vi "ini_sesion.vi"(8 "error in (no error)":errorcluster, 11 "p2p vst in":refnum<class "p2p vst.lvclass">) -> (0 "error out":errorcluster, 3 "p2p vst out":refnum<class "p2p vst.lvclass">)   [LabVIEW 2021, in "p2p vst.lvclass"]
uses:
  p2p vst.lvclass
  p2p vst.lvclass/p2p vst.ctl
  <instrlib>/niRFSG/niRFSG.llb/niRFSG Ref Clock Sources.ctl
  <vilib>/FPGAPlugInAG/PXIe-5785 (KU060)/niLvFpga_Open_PXIe-5785 (KU060).vi
  <vilib>/rvi/interface/common/dynamic/niFpgaDynamicAddResources.vi
  <vilib>/FPGAPlugInAG/Dynamic/niLvFpga_P2PGetEndpoint_Dynamic.vi
  <vilib>/Utility/error.llb/Error Cluster From Error Code.vi
  <vilib>/rvi/interface/common/niFpgaWaitOnOcc.vi
  <vilib>/rvi/errors/niLvFpgaAdjustHostInterfaceError.vi
  <vilib>/rvi/interface/nirviOpenFPGA/nirviOpenFPGA.xnode
  FPGA Bitfiles/P2P_Pulse.lvbitx
  <vilib>/rvi/interface/nirviMethod/nirviMethod.xnode
  <vilib>/rvi/interface/nirviReadWriteControl/nirviReadWriteControl.xnode
  <vilib>/FPGAPlugInAG/Dynamic/niLvFpga_ConfigureFifo_Dynamic.vi
  <vilib>/rvi/errors/niLvFpgaMergeErrorWithErrorCode.vi
  <vilib>/FPGAPlugInAG/Dynamic/niLvFpga_StopFifo_Dynamic.vi
  NiFpgaLv.dll
  <vilib>/rvi/interface/Simulation/niFpgaSimulationCallBeginRW.vi
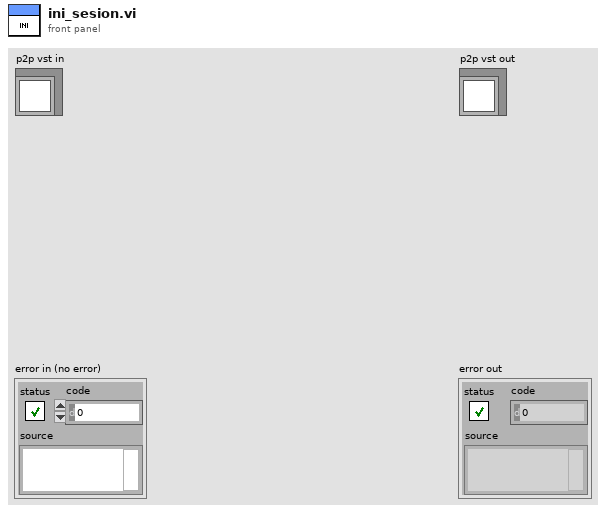
[diagram p1: front panel]
types:
  T1 = typedef "nirio_resource_hc.ctl" = tag
  T2 = typedef "niRFSG Ref Clock Sources.ctl" = string
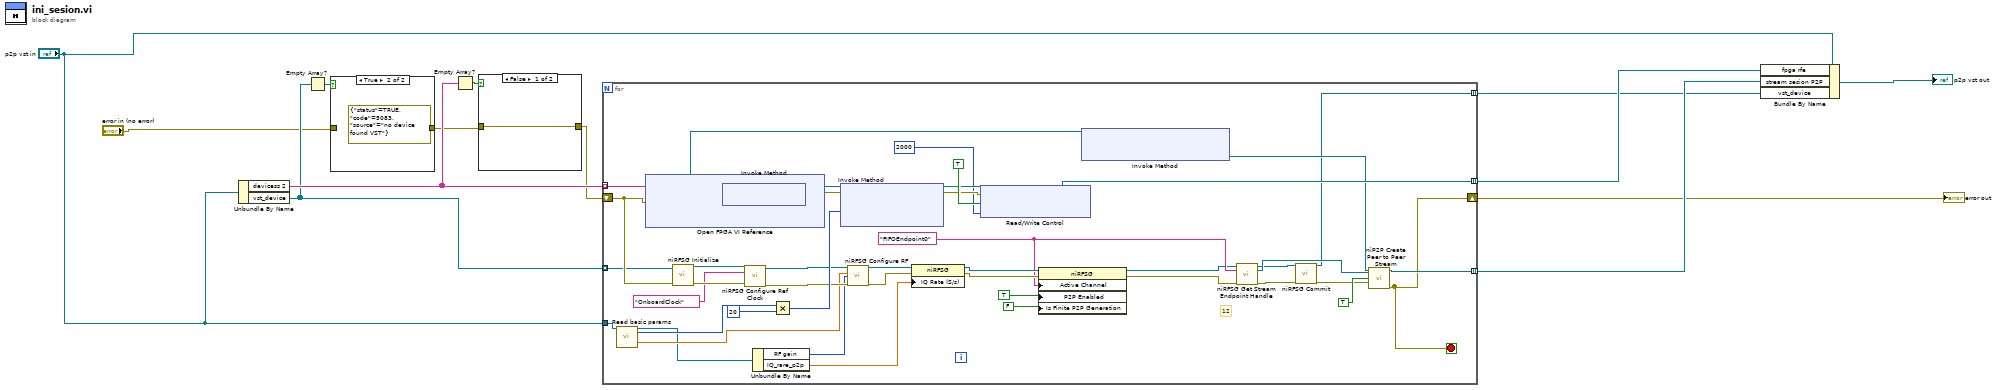
[diagram p0: block diagram]
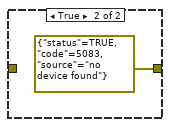
[diagram p3: hidden frame]
diagram:
  n1 = Unbundle By Name("p2p vst in") -> ("devicess 2"=w10:T1[], "vst_device"=w8:refnum<k15>[])
  n2 = Empty Array?(array=w8) -> (empty?=w9:bool)
  n3 = case shown="True" w9 {
    tunnel: [w14 errorcluster {"status"=TRUE, "code"=5083, "source"="no device found VST"} ("error in (no error)")] -> w7
    tunnel: "error in (no error)" -> [w14 _]
    frame False {
    }
    frame True {
    }
  }
  n4 = Empty Array?(array=w10) -> (empty?=w11:bool)
  n5 = case shown="False" w11 {
    tunnel: [w16 errorcluster {"status"=TRUE, "code"=5083, "source"="no device found"} ("error in (no error)")] -> w6
    tunnel: w7 -> [w16 _]
    frame False {
    }
    frame True {
    }
  }
  n6 = for {
    tunnel: [w46] -> w13 mode=indexing
    shift-right: [w40] -> w2
    shift-left: w6 -> [w48]
    tunnel: w10 -> [w52] mode=indexing
    tunnel: w8 -> [w44] mode=indexing
    tunnel: [w41] -> w12 mode=indexing
    tunnel: "p2p vst in" -> [w22]
    tunnel: [w18] -> w1 mode=indexing
    stop <- w40 stop-if-true
    w26 = "FIFOEndpoint0" ("format string")
    # "12"
    n7 = call-dynamic "Read basic params.vi"("device_type in"=w22) -> ("device_type out"=w19:refnum<class "p2p vst.lvclass">, "buffer size"=w21:u32, "center frequency (Hz)"=w20:dbl)  [unwired: 13 in, 3 out]
    n8 = xnode "Open FPGA VI Reference"("error in"=w48, "resource name"=w52) -> ("FPGA VI Reference Out"=w45:refnum<k20>, "error out"=w58:errorcluster)
    n9 = call <instrlib>:"niRFSG Initialize.vi"("resource name"=w44, "error in"=w48) -> ("instrument handle"=w51:refnum<k15>, "error out"=w50:errorcluster)  [unwired: 12 in]
    n10 = xnode "Invoke Method"("FPGA VI Reference In"=w45, "error in"=w58) -> ("FPGA VI Reference Out"=w56:refnum<k20>, "error out"=w57:errorcluster)
    n11 = call <instrlib>:"niRFSG Configure Ref Clock.vi"("instrument handle"=w51, "ref clock source"=T2 "OnboardClock", "error in"=w50) -> ("instrument handle out"=w37:refnum<k15>, "error out"=w36:errorcluster)  [unwired: 11 in]
    n12 = Unbundle By Name(w19) -> ("RF gain"=w35:i32, "IQ_rare_p2p"=w30:dbl)
    n13 = Multiply(x=w21, y=u32 20) -> (x*y=w60:u32)
    n14 = xnode "Invoke Method"("FPGA VI Reference In"=w56, "error in"=w57, "Requested Depth"=w60) -> ("FPGA VI Reference Out"=w54:refnum<k20>, "error out"=w53:errorcluster)  [unwired: 1 out]
    n15 = call <instrlib>:"niRFSG Configure RF.vi"("instrument handle"=w37, "frequency (Hz)"=w20, "power level (dBm)"=w35, "error in"=w36) -> ("instrument handle out"=w34:refnum<k15>, "error out"=w33:errorcluster)  [unwired: 10 in]
    n16 = property class="niRFSG"(reference=w34, error in=w33, "IQ Rate (S/s)"=w30) -> (reference out=w32:refnum<k15>, error out=w31:errorcluster)
    n17 = xnode "Read/Write Control"("FPGA VI Reference In"=w54, "error in"=w53, "reset system clock"=TRUE, "P2P empty room for runing"=u32 2000) -> ("FPGA VI Reference Out"=w46:refnum<k20>)  [unwired: 1 out]
    n18 = property class="niRFSG"(reference=w32, error in=w31, "Active Channel"=w26, "P2P Enabled"=TRUE ("Peer-to-Peer:Enabled"), "Is Finite P2P Generation"=FALSE ("Peer-to-Peer:Is Finite Generation")) -> (reference out=w25:refnum<k15>, error out=w24:errorcluster)
    n19 = xnode "Invoke Method"("FPGA VI Reference In"=w45) -> ("Writer"=w43:refnum<k20>)  [unwired: 1 in, 2 out]
    n20 = call <instrlib>:"niRFSG Get Stream Endpoint Handle.vi"("instrument handle"=w25, "stream endpoint"=w26, "error in"=w24) -> ("instrument handle out"=w29:refnum<k15>, "reader handle"=w47:refnum<k20>, "error out"=w28:errorcluster)  [unwired: 10 in]
    n21 = call <instrlib>:"niRFSG Commit.vi"("instrument handle"=w29, "error in"=w28) -> ("instrument handle out"=w18:refnum<k15>, "error out"=w27:errorcluster)  [unwired: 12 in]
    n22 = call <vilib>:"niP2P Create Peer to Peer Stream.vi"("writer"=w43, "reader"=w47, "enable stream (T)"=TRUE, "error in (no error)"=w27) -> ("stream session"=w41:refnum<k20>, "error out"=w40:errorcluster)  [unwired: 10 in]
  }
  "error out" <- w2
  n23 = Bundle By Name(cluster="p2p vst in", "fpga rfe"=w13, "stream sesion P2P"=w12, "vst_device"=w1) -> (→"p2p vst out":refnum<class "p2p vst.lvclass">)
